vi "Set Property.vi"(8 "error in (no error)":errorcluster, 9 "Data":variant, 10 "Key":string, 11 "Base Step in":refnum<class "Base Step.lvclass">) -> (0 "error out":errorcluster, 3 "Base Step out":refnum<class "Base Step.lvclass">)   [LabVIEW 2024, in "Ramses Sequencer.lvlib" / "Base Step.lvclass"]
uses:
  Base Step.lvclass
  Base Step.lvclass/Base Step.ctl
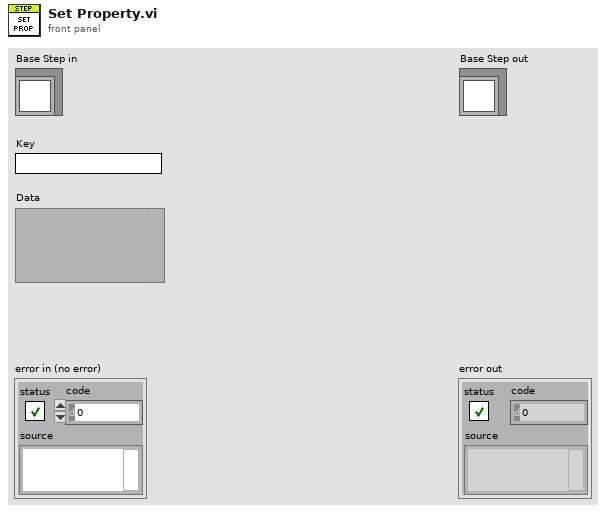
[diagram p1: front panel]
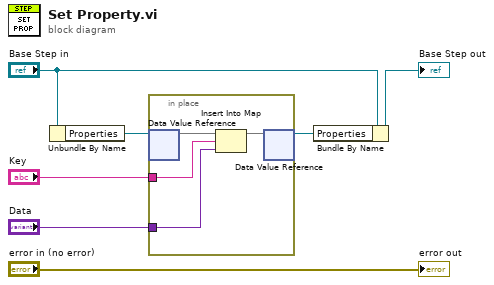
[diagram p0: block diagram]
diagram:
  n1 = Unbundle By Name("Base Step in") -> ("Properties"=w2:refnum<data-value>)
  n2 = in-place {
    in-place-border: "Key" -> [w11]
    in-place-border: "Data" -> [w10]
    n3 = in-place-dvr #1(w2) -> (w9:map{string, variant})  [unwired: 1 out]
    n4 = Insert Into Map(map in=w9, key=w11, value=w10) -> (map out=w8:map{string, variant})  [unwired: 2 out]
    n5 = in-place-dvr #1(w8) -> (w1:refnum<data-value>)  [unwired: 1 out]
  }
  n6 = Bundle By Name(cluster="Base Step in", "Properties"=w1) -> (→"Base Step out":refnum<class "Base Step.lvclass">)
  "error out" <- "error in (no error)"
